vi "test BOOL-2.vi"(11 "Test Case In":refnum<class "Build Sequence Test.lvclass">) -> (0 "error out":errorcluster, 3 "Test Case Out":refnum<class "Build Sequence Test.lvclass">)   [LabVIEW 2020, in "Build Sequence Test.lvclass"]
uses:
  Build Sequence Test.lvclass
  Build Sequence Test.lvclass/Build Sequence Test.ctl
  4993e8ee-a06a-463a-9684-69129f64d5ce.vi
  CANopen/CANopen.lvclass
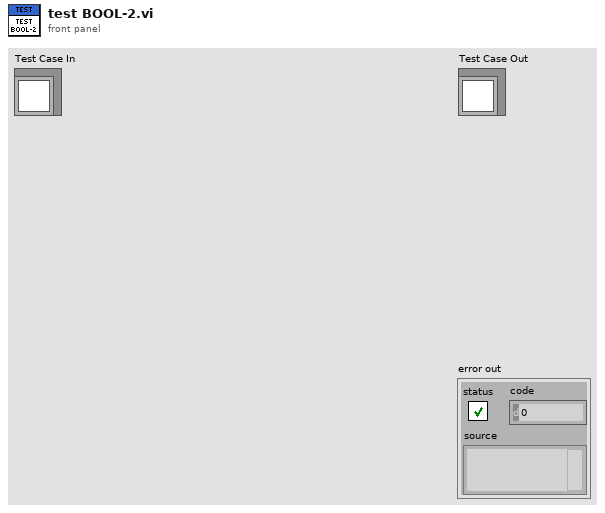
[diagram p1: front panel]
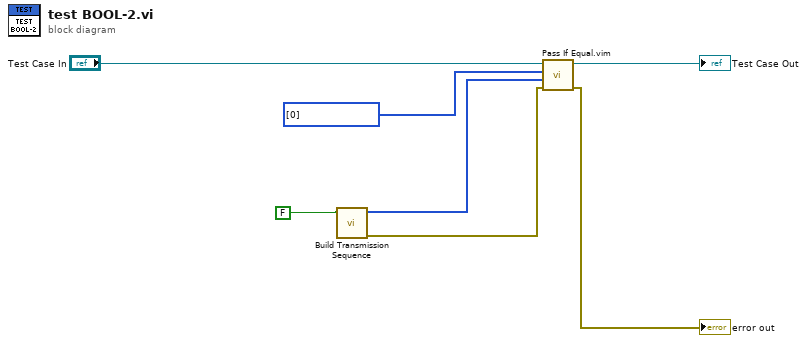
[diagram p0: block diagram]
diagram:
  n1 = call "Build Transmission Sequence.vi"("Data"=FALSE) -> ("error out"=w2:errorcluster, "Transmission Sequence"=w4:u8[])  [unwired: 9 in]
  n2 = call "Pass If Equal.vim"("error in (no error)"=w2, "Actual"=w4, "Expected"=u8[] [0] ("appended array"), "LUnit Test Case In"="Test Case In") -> ("error out"=→"error out":errorcluster, "LUnit Test Case Out"=→"Test Case Out":refnum<class "Build Sequence Test.lvclass">)  [unwired: 6 in]
